vi "3.2.vi"() -> ()   [LabVIEW 2014]
panel:
  out "# of iterations ouput":i32
  out "Current Number":dbl format="%#.0f"
  in  "number to match":dbl=50.0 min=0.0 max=1000.0 step=1.0 format="%#.0f"
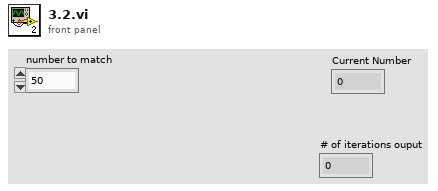
[diagram p1: front panel]
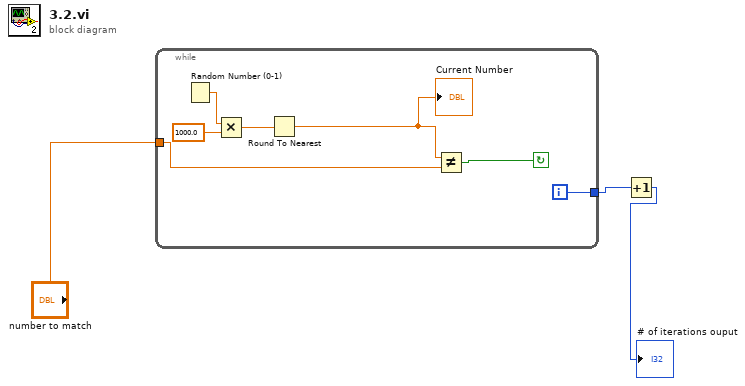
[diagram p0: block diagram]
diagram:
  n1 = while {
    tunnel: "number to match" -> [w9]
    tunnel: [w10] -> w2
    i -> [w10]
    stop <- w4 continue-if-true
    n2 = Random Number (0-1)() -> (number: 0 to 1=w7:dbl)
    n3 = Multiply(x=w7, y=1000.0) -> (x*y=w6:dbl)
    n4 = Round To Nearest(number=w6) -> (nearest integer value=w5:dbl)
    "Current Number" <- w5
    n5 = Not Equal?(x=w5, y=w9) -> (x != y?=w4:bool)
  }
  n6 = Increment(x=w2) -> (x+1=→"# of iterations ouput":i32)
